vi "Read Signal Samples to File.vi"() -> ()   [LabVIEW 2014]
uses:
  <vilib>/LabVIEW Universal Transcriptor/LabVIEW to Arduino Transcriptor/Transcriptors/System API/Serial println string.vi
  <vilib>/LabVIEW Universal Transcriptor/LabVIEW to Arduino Transcriptor/Transcriptors/System API/Serial print string.vi
  LabVIEW-Universal-Transcriptor-SD-Card-Library/File.lvclass
  <vilib>/LabVIEW Universal Transcriptor/LabVIEW Universal Transcriptor SD Card Library/LabVIEW Universal Transcriptor SD Card Library.lvlib
  <vilib>/LabVIEW Universal Transcriptor/LabVIEW to Arduino Transcriptor/Transcriptors/System API/System Serial Library Variables/System Serial Library Variables.lvlib
panel:
  out "String Buffer":string
  out "error out":errorcluster
  in  "Error In":errorcluster
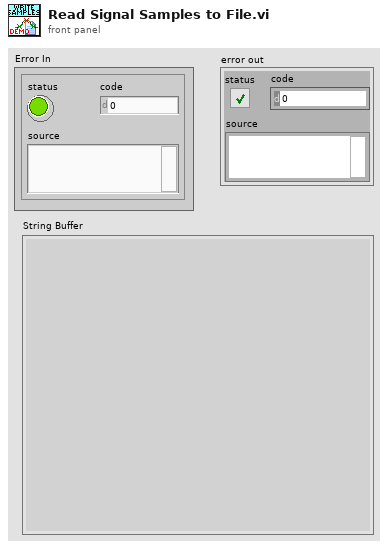
[diagram p1: front panel]
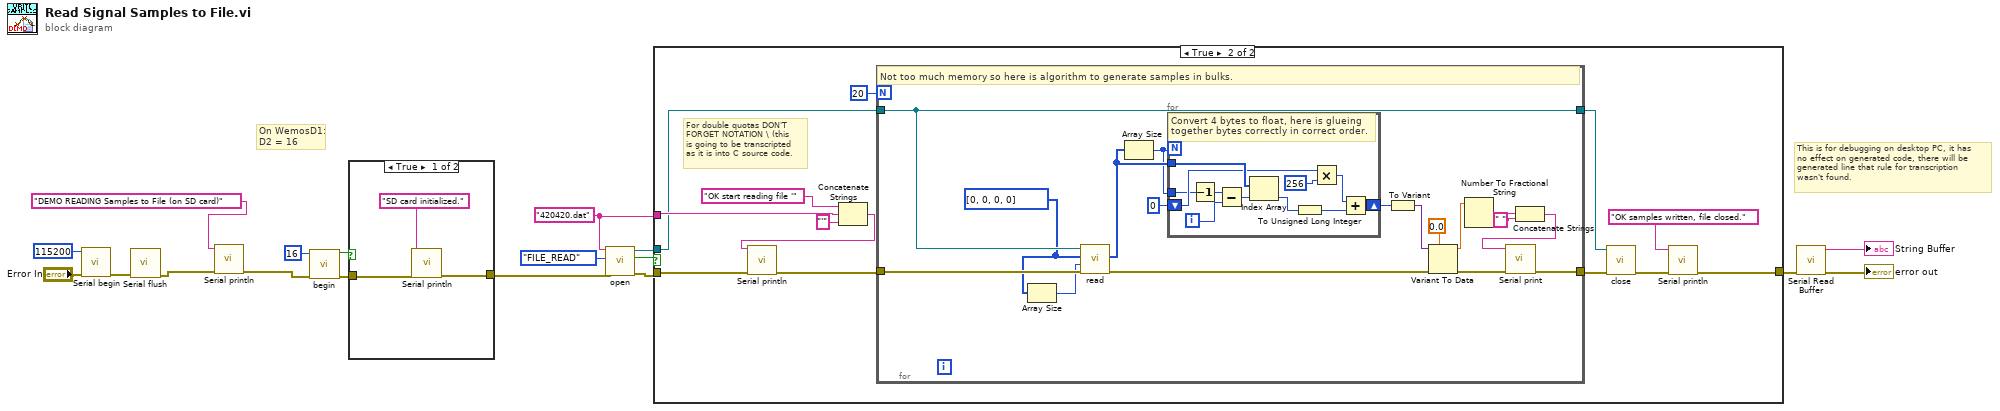
[diagram p0: block diagram]
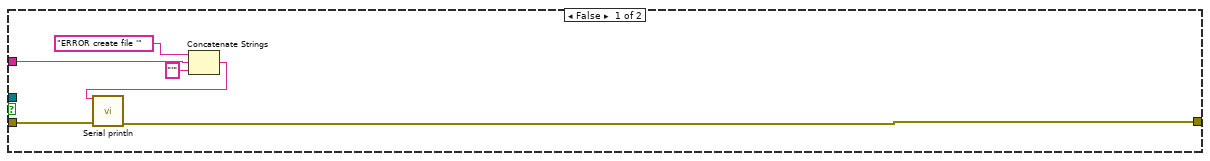
[diagram p2: hidden frame]
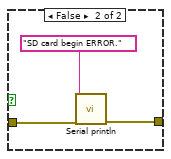
[diagram p3: hidden frame]
diagram:
  w7 = "420420.dat" ("filepath")
  # "On WemosD1:\nD2 = 16"
  # "This is for debugging on desktop PC, it has\nno effect on generated code, there will be\ngenerated line that rule for transcription\nwasn't found."
  n1 = call <vilib>:"Serial begin.vi"("Error In"="Error In", "speed (Bd)"=115200) -> ("Error Out"=w18:errorcluster)  [unwired: 9 in]
  n2 = call <vilib>:"Serial flush.vi"("Error In"=w18) -> ("Error Out"=w16:errorcluster)  [unwired: 10 in]
  n3 = call-poly <vilib>:"Serial println.vi"("Error In"=w16, "string in"="DEMO READING Samples to File (on SD card)") -> ("Error Out"=w14:errorcluster)  [unwired: 9 in]
  n4 = call <vilib>:"begin.vi"("Error In"=w14, "CS pin (optional)"=u8 16) -> ("Error Out"=w11:errorcluster, "success?"=w12:bool)  [unwired: 8 in]
  n5 = case shown="True" w12 {
    tunnel: w11 -> [w21 w24]
    tunnel: [w19 w22] -> w1
    frame True {
      n6 = call-poly <vilib>:"Serial println.vi"("Error In"=w21, "string in"="SD card initialized.") -> ("Error Out"=w19:errorcluster)  [unwired: 9 in]
    }
    frame False {
      n7 = call-poly <vilib>:"Serial println.vi"("Error In"=w24, "string in"="SD card begin ERROR.") -> ("Error Out"=w22:errorcluster)  [unwired: 9 in]
    }
  }
  n8 = call <vilib>:"open.vi"("Error In"=w1, "mode"=enum16{"FILE_READ", "FILE_WRITE"}."FILE_READ", "filepath"=w7) -> ("Error Out"=w9:errorcluster, "opened?"=w8:bool, "File out"=w6:refnum<class "File.lvclass">)  [unwired: 6 in]
  n9 = case shown="True" w8 {
    tunnel: w9 -> [w26 w40]
    tunnel: w7 -> [w30 w39]
    tunnel: [w25 w32] -> w5
    tunnel: w6 -> [_ w37]
    frame False {
      n10 = Concatenate Strings("ERROR create file '" ("string in"), w30, "'" ("string")) -> (w27:string)
      n11 = call-poly <vilib>:"Serial println.vi"("Error In"=w26, "string in"=w27) -> ("Error Out"=w25:errorcluster)  [unwired: 9 in]
    }
    frame True {
      # "For double quotas DON'T\nFORGET NOTATION \\ (this\nis going to be transcripted\nas it is into C source code."
      n12 = Concatenate Strings("OK start reading file '" ("string in"), w39, "'" ("string")) -> (w41:string)
      n13 = call-poly <vilib>:"Serial println.vi"("Error In"=w40, "string in"=w41) -> ("Error Out"=w38:errorcluster)  [unwired: 9 in]
      n14 = for {
        N: 20 -> [_]
        tunnel: w38 -> [w56]
        tunnel: w37 -> [w55]
        tunnel: [w55] -> w36
        tunnel: [w60] -> w31
        w54 = u8[] [0, 0, 0, 0] ("buffer")
        # "Not too much memory so here is algorithm to generate samples in bulks."
        n15 = Array Size(array=w54) -> (size(s)=w53:i32)
        n16 = call-dynamic "read.vi"("error in (no error)"=w56, "length"=w53, "buffer"=w54, "File in"=w55) -> ("error out"=w49:errorcluster, "buffer out"=w52:u8[])  [unwired: 6 in]
        n17 = Array Size(array=w52) -> (size(s)=w44:i32)
        n18 = for {
          N: w44 -> [_]
          tunnel: w52 -> [w71]
          shift-right: [w66] -> w50
          shift-left: u32 0 ("element") -> [w70]
          tunnel: w44 -> [w65]
          i -> [w64]
          # "Convert 4 bytes to float, here is glueing together bytes correctly in correct order."
          n19 = Decrement(x=w65) -> (x-1=w63:i32)
          n20 = Subtract(x=w63, y=w64) -> (x-y=w62:i32)
          n21 = Index Array(array=w71, index=w62) -> (element=w67:u8)
          n22 = To Unsigned Long Integer(number=w67) -> (unsigned 32bit integer=w61:u32)
          n23 = Multiply(x=w70, y=u32 256) -> (x*y=w68:u32)
          n24 = Add(x=w68, y=w61) -> (x+y=w66:u32)
        }
        n25 = To Variant(anything=w50) -> (Variant=w47:variant)
        n26 = Variant To Data(error in=w49, type=sgl 0.0, Variant=w47) -> (data=w46:sgl, error out=w48:errorcluster)
        n27 = Number To Fractional String(number=w46) -> (F-format string=w58:string)  [unwired: 3 in]
        n28 = Concatenate Strings(w58, " " ("element")) -> (w57:string)
        n29 = call-poly <vilib>:"Serial print.vi"("Error In"=w48, "string in"=w57) -> ("Error Out"=w60:errorcluster)  [unwired: 9 in]
      }
      n30 = call-dynamic "close.vi"("error in (no error)"=w31, "File in"=w36) -> ("error out"=w33:errorcluster)  [unwired: 9 in]
      n31 = call-poly <vilib>:"Serial println.vi"("Error In"=w33, "string in"="OK samples written, file closed.") -> ("Error Out"=w32:errorcluster)  [unwired: 9 in]
    }
  }
  n32 = call <vilib>:"Serial Read Buffer.vi"("Error In"=w5) -> ("Error Out"=→"error out":errorcluster, "String Buffer"=→"String Buffer":string)  [unwired: 9 in]
